vi "Read Dashboard Variables.vi"() -> ()   [LabVIEW 2019]
uses:
  <vilib>/Rock Robotics/Network Tables/NT Read Number.vi
  Framework/Robot Global Data.vi
  <vilib>/Rock Robotics/Network Tables/NT Read String.vi
  <vilib>/Rock Robotics/Network Tables/NT Read Variant.vi
panel:
  out "Blue Calibration":cluster{"R":dbl, "G":dbl, "B":dbl}={"R"=0.143, "G"=0.427, "B"=0.429}
  out "Green Calibration":cluster{"R":dbl, "G":dbl, "B":dbl}={"R"=0.197, "G"=0.561, "B"=0.24}
  out "Red Calibration":cluster{"R":dbl, "G":dbl, "B":dbl}={"R"=0.561, "G"=0.323, "B"=0.114}
  out "Yellow Calibration":cluster{"R":dbl, "G":dbl, "B":dbl}={"R"=0.361, "G"=0.524, "B"=0.113}
  out "Path":string
  out "MaxSpeedSlow":dbl=0.6
  out "Pivot Left":dbl=0.3
  out "Pivot right":dbl=0.4
  out "Intake Set Point":dbl=1.0
  out "Intake Duration":dbl=0.5
  out "Shooter Set Point":dbl=1.0
  out "Shooter Duration":dbl=0.5
  out "Transfer Set Point":dbl=0.6
  out "Transfer Duration":dbl=0.5
  out "Control Panel Set Point":dbl=0.6
  out "Control Panel Duration":dbl=5.5
  out "Control Panel Color Set Point":dbl=0.3
  out "Control Panel Color Duration":dbl=4.0
  out "MaxDrive":dbl(slide)=1.0 min=0.0 max=1.0 step=0.01 scale=0.0..1.0
  out "DriveK":dbl(slide)=0.5 min=0.0 max=1.0 step=0.05 scale=0.0..1.0
  out "Limelight Goal Area":dbl(slide)=1.91 min=0.1 max=2.5 step=0.25 scale=0.0..2.5
  out "MinSteerCommand":dbl(slide)=0.2717391304347826 min=0.0 max=0.5 step=0.05 scale=0.0..0.5
  out "SteeringK":dbl(slide)=0.025362318840579712 min=0.0 max=0.25 step=0.01 scale=0.0..0.25
  out "AimDeadband":dbl=0.1 min=0.0 max=10.0 step=0.25
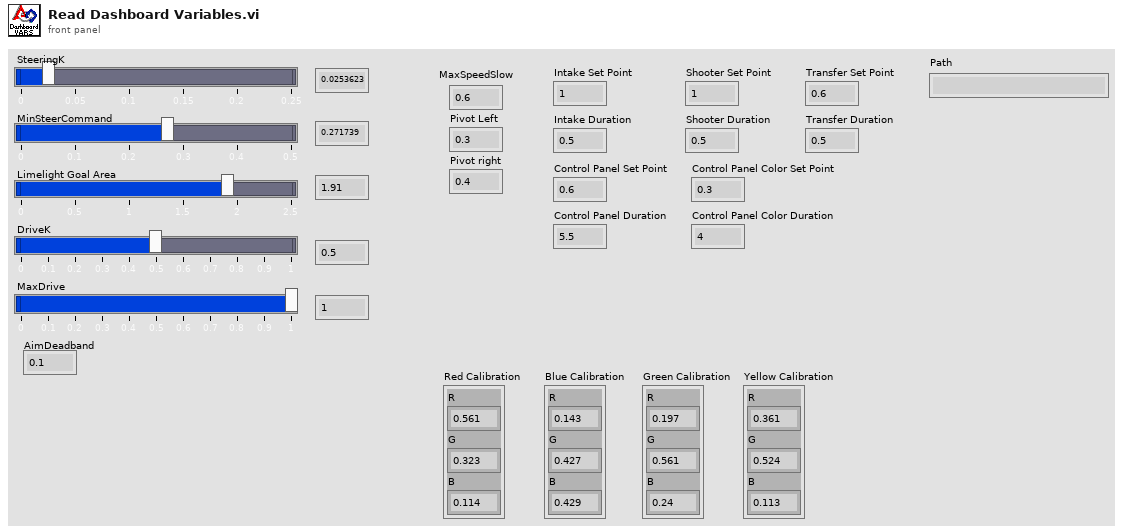
[diagram p1: front panel]
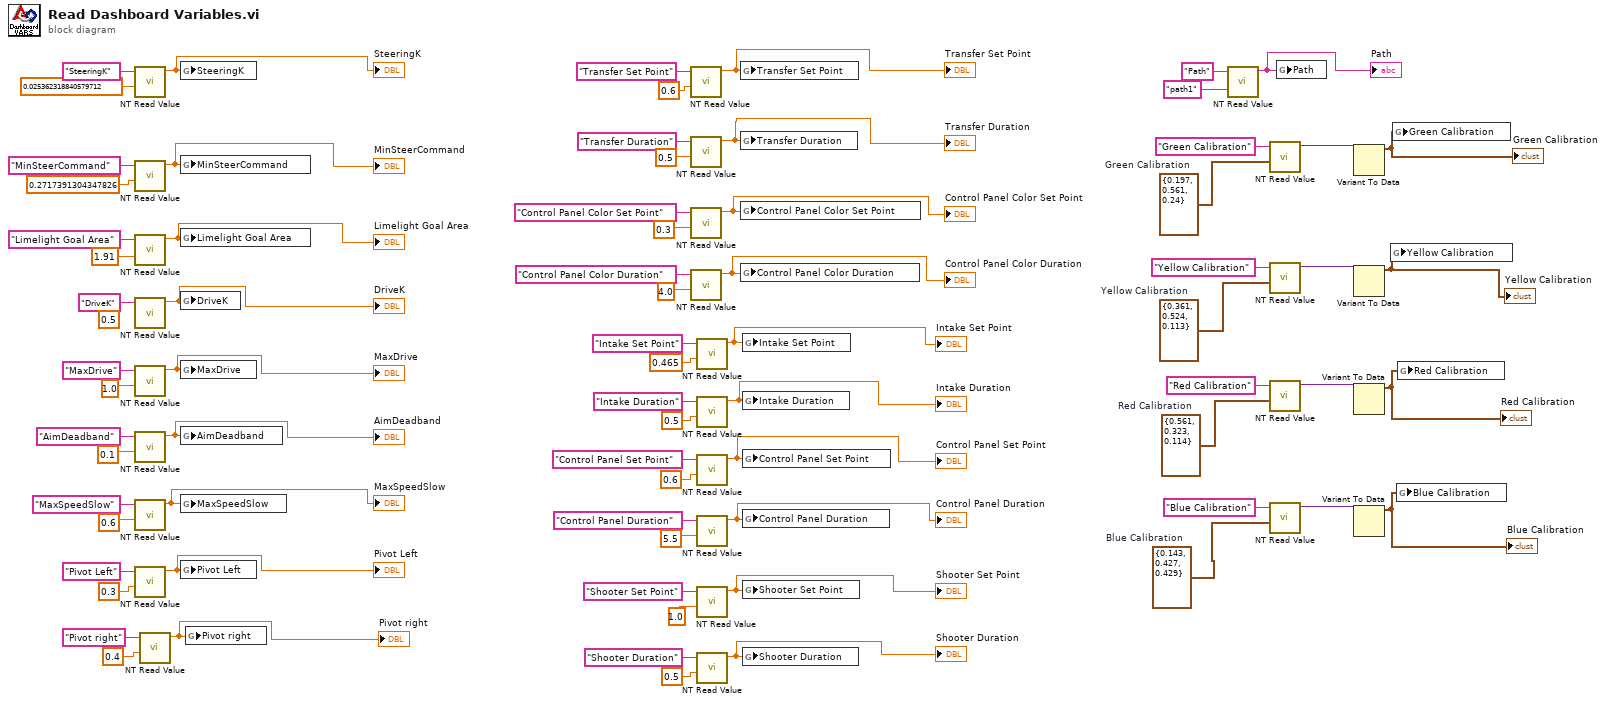
[diagram p0: block diagram]
diagram:
  w3 = cluster{"R":dbl, "G":dbl, "B":dbl} {"R"=0.143, "G"=0.427, "B"=0.429}  # Blue Calibration
  w2 = cluster{"R":dbl, "G":dbl, "B":dbl} {"R"=0.561, "G"=0.323, "B"=0.114}  # Red Calibration
  w1 = cluster{"R":dbl, "G":dbl, "B":dbl} {"R"=0.361, "G"=0.524, "B"=0.113}  # Yellow Calibration
  w15 = cluster{"R":dbl, "G":dbl, "B":dbl} {"R"=0.197, "G"=0.561, "B"=0.24}  # Green Calibration
  (unwired) 0.5 ("DriveK")
  n1 = call-poly <vilib>:"NT Read Value.vi"("Default Value"=0.025362318840579712 ("SteeringK"), "Name"="SteeringK") -> ("Numeric"=w38:dbl)  [unwired: 8 in, 1 out]
  "SteeringK" <- w38
  n2 = call-poly <vilib>:"NT Read Value.vi"("Default Value"=0.2717391304347826 ("MinSteerCommand"), "Name"="MinSteerCommand") -> ("Numeric"=w21:dbl)  [unwired: 8 in, 1 out]
  "MinSteerCommand" <- w21
  n3 = call-poly <vilib>:"NT Read Value.vi"("Default Value"=1.91 ("Limelight Goal Area"), "Name"="Limelight Goal Area") -> ("Numeric"=w37:dbl)  [unwired: 8 in, 1 out]
  "Limelight Goal Area" <- w37
  n4 = call-poly <vilib>:"NT Read Value.vi"("Name"="DriveK") -> ("Numeric"=w36:dbl)  [unwired: 9 in, 1 out]
  "DriveK" <- w36
  n5 = call-poly <vilib>:"NT Read Value.vi"("Default Value"=1.0 ("MaxDrive"), "Name"="MaxDrive") -> ("Numeric"=w35:dbl)  [unwired: 8 in, 1 out]
  "MaxDrive" <- w35
  n6 = call-poly <vilib>:"NT Read Value.vi"("Default Value"=0.1 ("AimDeadband"), "Name"="AimDeadband") -> ("Numeric"=w34:dbl)  [unwired: 8 in, 1 out]
  "AimDeadband" <- w34
  n7 = call-poly <vilib>:"NT Read Value.vi"("Default Value"=0.6 ("MaxSpeedSlow"), "Name"="MaxSpeedSlow") -> ("Numeric"=w33:dbl)  [unwired: 8 in, 1 out]
  "MaxSpeedSlow" <- w33
  n8 = call-poly <vilib>:"NT Read Value.vi"("Default Value"=0.3 ("Pivot Left"), "Name"="Pivot Left") -> ("Numeric"=w32:dbl)  [unwired: 8 in, 1 out]
  "Pivot Left" <- w32
  n9 = call-poly <vilib>:"NT Read Value.vi"("Default Value"=0.4 ("Pivot right"), "Name"="Pivot right") -> ("Numeric"=w31:dbl)  [unwired: 8 in, 1 out]
  "Pivot right" <- w31
  n10 = global write "Robot Global Data.vi" "SteeringK"(w38) -> ()
  n11 = global write "Robot Global Data.vi" "MinSteerCommand"(w21) -> ()
  n12 = global write "Robot Global Data.vi" "Limelight Goal Area"(w37) -> ()
  n13 = global write "Robot Global Data.vi" "DriveK"(w36) -> ()
  n14 = global write "Robot Global Data.vi" "MaxDrive"(w35) -> ()
  n15 = global write "Robot Global Data.vi" "AimDeadband"(w34) -> ()
  n16 = global write "Robot Global Data.vi" "MaxSpeedSlow"(w33) -> ()
  n17 = global write "Robot Global Data.vi" "Pivot Left"(w32) -> ()
  n18 = global write "Robot Global Data.vi" "Pivot right"(w31) -> ()
  n19 = call-poly <vilib>:"NT Read Value.vi"("Default Value"=0.6 ("Transfer Set Point"), "Name"="Transfer Set Point") -> ("Numeric"=w25:dbl)  [unwired: 8 in, 1 out]
  "Transfer Set Point" <- w25
  n20 = call-poly <vilib>:"NT Read Value.vi"("Default Value"=0.5 ("Transfer Duration"), "Name"="Transfer Duration") -> ("Numeric"=w24:dbl)  [unwired: 8 in, 1 out]
  "Transfer Duration" <- w24
  n21 = call-poly <vilib>:"NT Read Value.vi"("Default Value"=0.3 ("Control Panel Color Set Point"), "Name"="Control Panel Color Set Point") -> ("Numeric"=w23:dbl)  [unwired: 8 in, 1 out]
  "Control Panel Color Set Point" <- w23
  n22 = call-poly <vilib>:"NT Read Value.vi"("Default Value"=4.0 ("Control Panel Color Duration"), "Name"="Control Panel Color Duration") -> ("Numeric"=w22:dbl)  [unwired: 8 in, 1 out]
  "Control Panel Color Duration" <- w22
  n23 = call-poly <vilib>:"NT Read Value.vi"("Default Value"=0.465 ("Intake Set Point"), "Name"="Intake Set Point") -> ("Numeric"=w20:dbl)  [unwired: 8 in, 1 out]
  "Intake Set Point" <- w20
  n24 = call-poly <vilib>:"NT Read Value.vi"("Default Value"=0.5 ("Intake Duration"), "Name"="Intake Duration") -> ("Numeric"=w30:dbl)  [unwired: 8 in, 1 out]
  "Intake Duration" <- w30
  n25 = call-poly <vilib>:"NT Read Value.vi"("Default Value"=0.6 ("Control Panel Set Point"), "Name"="Control Panel Set Point") -> ("Numeric"=w29:dbl)  [unwired: 8 in, 1 out]
  "Control Panel Set Point" <- w29
  n26 = call-poly <vilib>:"NT Read Value.vi"("Default Value"=5.5 ("Control Panel Duration"), "Name"="Control Panel Duration") -> ("Numeric"=w28:dbl)  [unwired: 8 in, 1 out]
  "Control Panel Duration" <- w28
  n27 = call-poly <vilib>:"NT Read Value.vi"("Default Value"=1.0 ("Shooter Set Point"), "Name"="Shooter Set Point") -> ("Numeric"=w27:dbl)  [unwired: 8 in, 1 out]
  "Shooter Set Point" <- w27
  n28 = call-poly <vilib>:"NT Read Value.vi"("Default Value"=0.5 ("Shooter Duration"), "Name"="Shooter Duration") -> ("Numeric"=w26:dbl)  [unwired: 8 in, 1 out]
  "Shooter Duration" <- w26
  n29 = global write "Robot Global Data.vi" "Transfer Set Point"(w25) -> ()
  n30 = global write "Robot Global Data.vi" "Transfer Duration"(w24) -> ()
  n31 = global write "Robot Global Data.vi" "Control Panel Color Set Point"(w23) -> ()
  n32 = global write "Robot Global Data.vi" "Control Panel Color Duration"(w22) -> ()
  n33 = global write "Robot Global Data.vi" "Intake Set Point"(w20) -> ()
  n34 = global write "Robot Global Data.vi" "Intake Duration"(w30) -> ()
  n35 = global write "Robot Global Data.vi" "Control Panel Set Point"(w29) -> ()
  n36 = global write "Robot Global Data.vi" "Control Panel Duration"(w28) -> ()
  n37 = global write "Robot Global Data.vi" "Shooter Set Point"(w27) -> ()
  n38 = global write "Robot Global Data.vi" "Shooter Duration"(w26) -> ()
  n39 = call-poly <vilib>:"NT Read Value.vi"("Default Value"="path1", "Name"="Path") -> ("String"=w17:string)  [unwired: 8 in, 1 out]
  "Path" <- w17
  n40 = call-poly <vilib>:"NT Read Value.vi"("Default Value"=w15, "Name"="Green Calibration") -> ("Variant"=w14:variant)  [unwired: 8 in, 1 out]
  n41 = call-poly <vilib>:"NT Read Value.vi"("Default Value"=w1, "Name"="Yellow Calibration") -> ("Variant"=w12:variant)  [unwired: 8 in, 1 out]
  n42 = call-poly <vilib>:"NT Read Value.vi"("Default Value"=w2, "Name"="Red Calibration") -> ("Variant"=w9:variant)  [unwired: 8 in, 1 out]
  n43 = call-poly <vilib>:"NT Read Value.vi"("Default Value"=w3, "Name"="Blue Calibration") -> ("Variant"=w8:variant)  [unwired: 8 in, 1 out]
  n44 = global write "Robot Global Data.vi" "Path"(w17) -> ()
  n45 = Variant To Data(Variant=w14) -> (data=w13:cluster{"R":dbl, "G":dbl, "B":dbl})  [unwired: 2 in, 1 out]
  "Green Calibration" <- w13
  n46 = Variant To Data(Variant=w12) -> (data=w6:cluster{"R":dbl, "G":dbl, "B":dbl})  [unwired: 2 in, 1 out]
  "Yellow Calibration" <- w6
  n47 = Variant To Data(Variant=w9) -> (data=w5:cluster{"R":dbl, "G":dbl, "B":dbl})  [unwired: 2 in, 1 out]
  "Red Calibration" <- w5
  n48 = Variant To Data(Variant=w8) -> (data=w4:cluster{"R":dbl, "G":dbl, "B":dbl})  [unwired: 2 in, 1 out]
  "Blue Calibration" <- w4
  n49 = global write "Robot Global Data.vi" "Yellow Calibration"(w6) -> ()
  n50 = global write "Robot Global Data.vi" "Green Calibration"(w13) -> ()
  n51 = global write "Robot Global Data.vi" "Blue Calibration"(w4) -> ()
  n52 = global write "Robot Global Data.vi" "Red Calibration"(w5) -> ()
